vi "SetParam.vi"(8 "error in (no error)":errorcluster caption="entrée d'erreur (pas d'erreur)", 10 "fetch_rcv1":T1={"subset"="all", "download_if_missing"=TRUE, "random_state"=0, "shuffle"=TRUE, "Returns"="Data"} {"random_state" min=-1}, 11 "Rcv1.lvclass":refnum<class "Rcv1.lvclass">) -> (0 "error out":errorcluster caption="sortie d'erreur", 3 "Rcv1.lvclass":refnum<class "Rcv1.lvclass">)   [LabVIEW 2020, in "Rcv1.lvclass"]
doc: "Set Parameters"
uses:
  Rcv1.lvclass
  Rcv1.lvclass/Rcv1.ctl
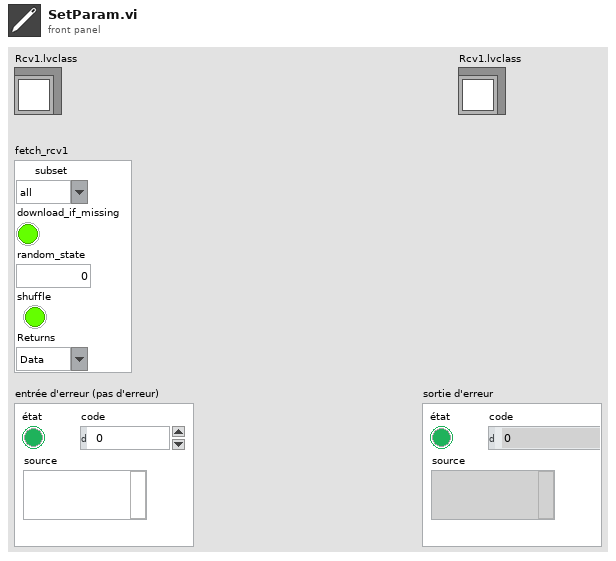
[diagram p1: front panel]
types:
  T1 = cluster{"subset":string, "download_if_missing":bool, "random_state":i32, "shuffle":bool, "Returns":string}
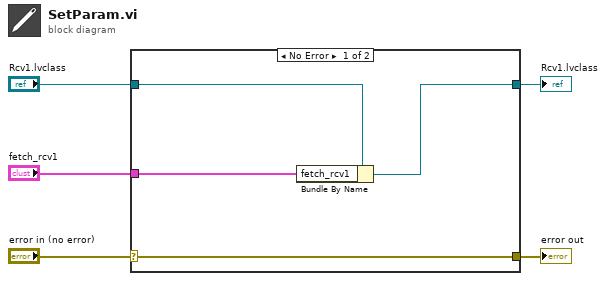
[diagram p0: block diagram]
diagram:
  n1 = case shown="No Error" "error in (no error)" {
    selector: "error in (no error)" -> [w9 w10]
    tunnel: [w9 w10] -> w4
    tunnel: [w7 w11] -> w2
    tunnel: "Rcv1.lvclass" -> [w8 w11]
    tunnel: "fetch_rcv1" -> [w6 _]
    frame No Error {
      n2 = Bundle By Name(cluster=w8, "fetch_rcv1"=w6) -> (w7:refnum<class "Rcv1.lvclass">)
    }
    frame Error {
    }
  }
  "error out" <- w4
  "Rcv1.lvclass" <- w2
